vi "Test Create Logger with Queue Sink.vi"(11 "Test Case In":refnum<class "Queue Sink.lvclass">) -> (0 "error out":errorcluster, 3 "Test Case Out":refnum<class "Queue Sink.lvclass">)   [LabVIEW 2020, in "Queue Sink.lvclass"]
uses:
  Queue Sink.lvclass
  C:/Program Files (x86)/National Instruments/LabVIEW 2020/vi.lib/Astemes/LUnit/Test Case.lvclass
  Source/Type Defs/Debug Level.ctl
  <vilib>/Astemes/LUnit/Test Case.lvclass/Test Case.ctl
  186b7594-36c3-475d-9f56-112695fdc62a.vi
  9f417576-4e54-4520-bbfc-3f0305dac5bd.vi
  abc007d3-7e1b-4fc8-9ad7-ed682a564c3c.vi
  <vilib>/Astemes/LUnit/Core/LUnit Test Case/Private/Append Pass Result.vi
  <vilib>/Astemes/LUnit/Core/LUnit Test Case/Private/Append Fail Result.vi
  186b7594-36c3-475d-9f56-112695fdc62a.vi/9c5d11cd-9439-4240-a1ee-d9baace9c924.vi
  9f417576-4e54-4520-bbfc-3f0305dac5bd.vi/9c5d11cd-9439-4240-a1ee-d9baace9c924.vi
  abc007d3-7e1b-4fc8-9ad7-ed682a564c3c.vi/9c5d11cd-9439-4240-a1ee-d9baace9c924.vi
  <vilib>/Astemes/LUnit/Core/LUnit Test Case/Private/Run In UI.vi
  <vilib>/Utility/error.llb/Clear Errors.vi
  Source/Sinks/Queue Sink/Queue Sink.lvclass
  C:/Users/hughe_cx/Documents/05_repos/LVLog/Source/Sinks/Sink/Sink.lvclass
  Queue Sink.lvclass/Queue Sink.ctl
  Source/LV Log.lvlib
  Source/Logger/Logger.lvclass
  <vilib>/Astemes/LUnit/Test Case.lvclass
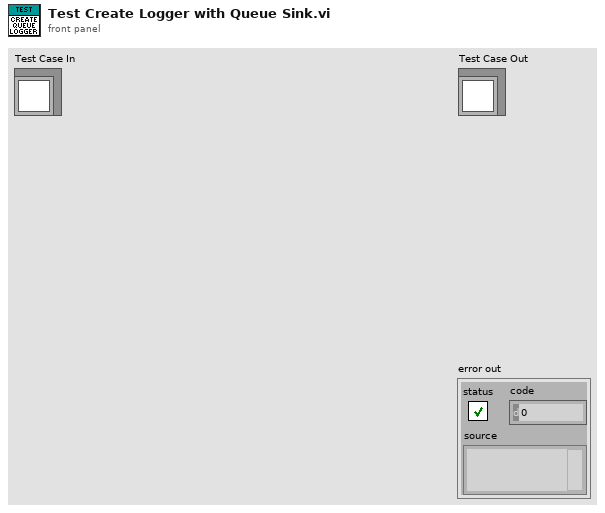
[diagram p1: front panel]
types:
  T1 = typedef "LV Log.lvlib/Debug Level.ctl" = enum16{"DEFAULT", "DEBUG", "INFO", "WARN", "ERROR", "FATAL"}
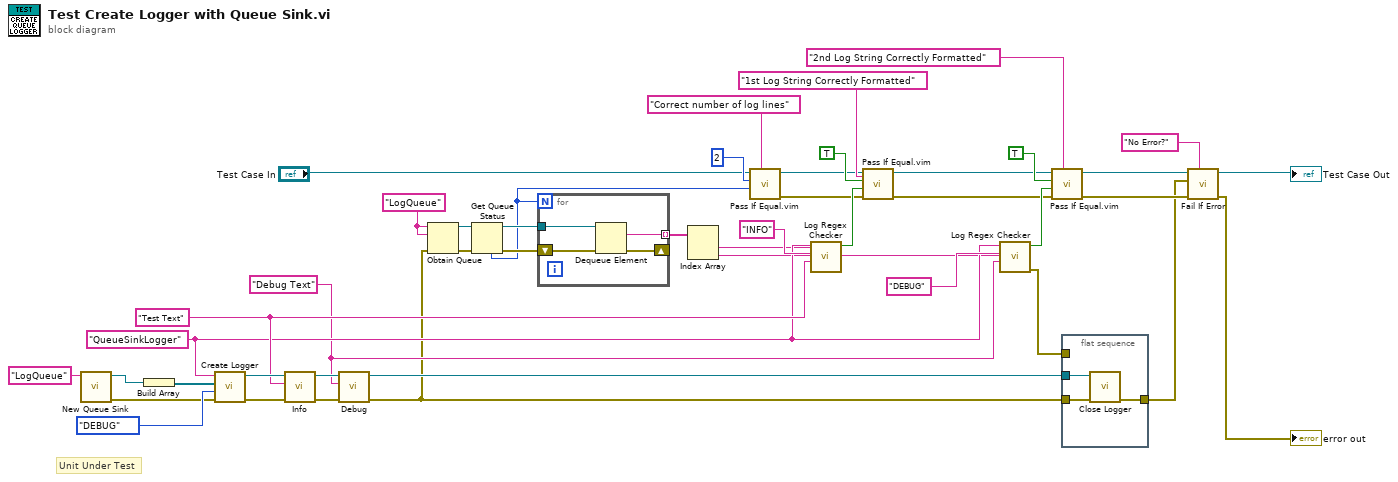
[diagram p0: block diagram]
diagram:
  w9 = "LogQueue" ("name (unnamed)")
  w32 = "Debug Text" ("Log Text")
  w41 = "Test Text" ("Log Text")
  w33 = "QueueSinkLogger" ("Name")
  # "Unit Under Test"
  n1 = call "New Queue Sink.vi"("Queue Name"="LogQueue") -> ("error out"=w13:errorcluster, "Queue Sink out"=w12:refnum<class "Queue Sink.lvclass">)  [unwired: 9 in]
  n2 = Build Array(w12) -> (w22:refnum<class "Queue Sink.lvclass">[])
  n3 = call "Create Logger.vi"("error in (no error)"=w13, "Debug Level (Default)"=Debug_Level."DEBUG" ("Debug Level in"), "Sinks (Default)"=w22, "Name"=w33) -> ("error out"=w45:errorcluster, "Logger out"=w44:refnum<class "Logger.lvclass">)  [unwired: 6 in]
  n4 = call "Info.vi"("error in (no error)"=w45, "Log Text"=w41, "Logger in"=w44) -> ("error out"=w40:errorcluster, "Logger out"=w39:refnum<class "Logger.lvclass">)  [unwired: 6 in, 1 out]
  n5 = call "Debug.vi"("error in (no error)"=w40, "Log Text"=w32, "Logger in"=w39) -> ("error out"=w1:errorcluster, "Logger out"=w20:refnum<class "Logger.lvclass">)  [unwired: 6 in, 1 out]
  n6 = Obtain Queue(name (unnamed)=w9, element data type=w9, error in (no error)=w1) -> (queue out=w5:refnum<queue>, error out=w6:errorcluster)  [unwired: 2 in, 1 out]
  n7 = Get Queue Status(queue=w5, error in (no error)=w6) -> (queue out=w8:refnum<queue>, error out=w7:errorcluster, # elements in queue=w4:i32)  [unwired: 1 in, 5 out]
  n8 = for {
    N: w4 -> [_]
    shift-right: [w47] -> _
    shift-left: w7 -> [w49]
    tunnel: w8 -> [w48]
    tunnel: [w46] -> w3 mode=indexing
    n9 = Dequeue Element(queue=w48, error in (no error)=w49) -> (element=w46:string, error out=w47:errorcluster)  [unwired: 1 in, 2 out]
  }
  n10 = Index Array(array=w3) -> (element #1=w31:string, element #2=w30:string)  [unwired: 2 in]
  n11 = call "Pass If Equal.vim"("Description"="Correct number of log lines", "Actual"=w4, "Expected"=2, "LUnit Test Case In"="Test Case In") -> ("error out"=w23:errorcluster, "LUnit Test Case Out"=w27:refnum<class "Queue Sink.lvclass">)  [unwired: 6 in]
  n12 = call "Log Regex Checker.vi"("Log String"=w31, "Expected Log Text (Any)"=w41, "Expected Log Level (Any)"="INFO", "Expected Logger Name (Any)"=w33) -> ("Math Found"=w37:bool)  [unwired: 5 in, 2 out]
  n13 = call "Pass If Equal.vim"("Description"="1st Log String Correctly Formatted", "error in (no error)"=w23, "Actual"=w37, "Expected"=TRUE, "LUnit Test Case In"=w27) -> ("error out"=w24:errorcluster, "LUnit Test Case Out"=w29:refnum<class "Queue Sink.lvclass">)  [unwired: 5 in]
  n14 = call "Log Regex Checker.vi"("Log String"=w30, "Expected Log Text (Any)"=w32, "Expected Log Level (Any)"="DEBUG", "Expected Logger Name (Any)"=w33) -> ("error out"=w2:errorcluster, "Math Found"=w36:bool)  [unwired: 5 in, 1 out]
  n15 = call "Pass If Equal.vim"("Description"="2nd Log String Correctly Formatted", "error in (no error)"=w24, "Actual"=w36, "Expected"=TRUE, "LUnit Test Case In"=w29) -> ("error out"=w25:errorcluster, "LUnit Test Case Out"=w28:refnum<class "Queue Sink.lvclass">)  [unwired: 5 in]
  n16 = flat-sequence {
    tunnel: w1 -> [w52]
    tunnel: w20 -> [w51]
    tunnel: [w50] -> w19
    tunnel: w2 -> [_]
    frame #0 {
      n17 = call "Close Logger.vi"("error in (no error)"=w52, "Logger in"=w51) -> ("error out"=w50:errorcluster)  [unwired: 9 in]
    }
  }
  n18 = call <vilib>:"Fail If Error.vi"("Description"="No Error?", "error in (no error)"=w25, "Assert error"=w19, "LUnit Test Case In"=w28) -> ("error out"=→"error out":errorcluster, "LUnit Test Case Out"=→"Test Case Out":refnum<class "Queue Sink.lvclass">)  [unwired: 6 in]
